vi "Initialize_Kate_Module.vi"(8 "Error In":errorcluster, 11 "UI Controls Refnum":T1) -> (0 "Error Out":errorcluster)   [LabVIEW 2012]
doc: "SciScan 1.2 160622"
uses:
  Custom Control and Typedefs/UI Controls Refnum.ctl
  Custom Control and Typedefs/ChannelSelector_for_PosSave.ctl
  Custom Controls/PositionSaveMod.ctl
  Custom Control and Typedefs/Overlay Control.ctl
  CommonResource VIs/UI Control and Indicator properties_Commands.ctl
  Image Validity FGV_Commands.ctl
  Custom Controls/MAIN Image panel tab Control type def.ctl
  Custom Controls/MAIN Image panel reso tab Control type def.ctl
  Chnl_2_tab_Commands.ctl
  GFG/GFG library.lvlib
panel:
  # "Red (Current Image)"
  # "Green (Saved Image)"
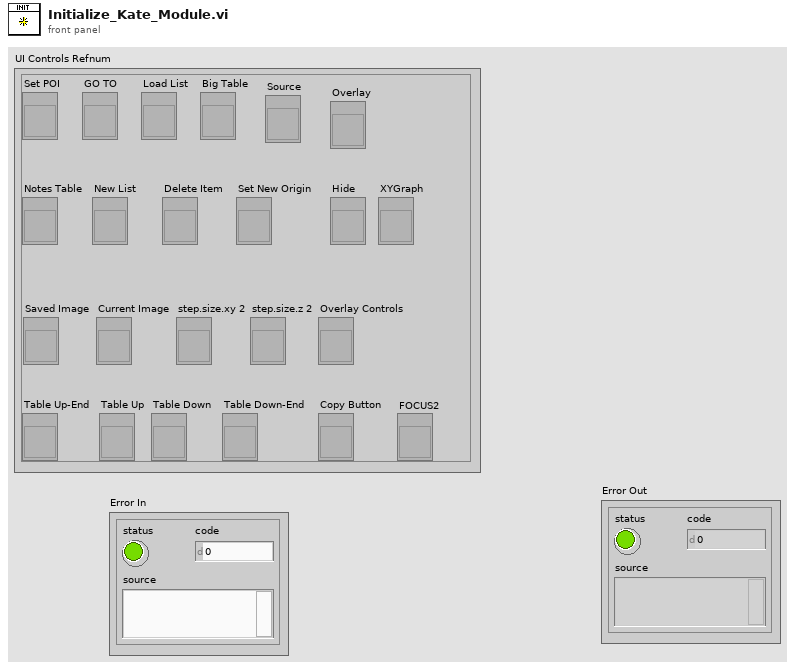
[diagram p1: front panel]
types:
  T1 = typedef "UI Controls Refnum.ctl" = cluster{"GO TO":refnum<vi>, "Load List":refnum<vi>, "Big Table":refnum<vi>, "Notes Table":refnum<vi>, "New List":refnum<vi>, "Delete Item":refnum<vi>, "Set New Origin":refnum<vi>, "Set POI":refnum<vi>, "Saved Image":refnum<vi>, "Current Image":refnum<vi>, "step.size.xy 2":refnum<vi>, "step.size.z 2":refnum<vi>, "Source":refnum<vi>, "Table Up-End":refnum<vi>, "Table Up":refnum<vi>, "Table Down":refnum<vi>, "Table Down-End":refnum<vi>, "Copy Button":refnum<vi>, "Hide":refnum<vi>, "Overlay Controls":refnum<vi>, "Overlay":refnum<vi>, "XYGraph":refnum<vi>, "FOCUS2":refnum<vi>}
  T2 = typedef "Image Validity FGV_Commands.ctl" = enum16{"Set validity status", "Get Validity status"}
  T3 = typedef "UI Control and Indicator properties_Commands.ctl" = enum16{"Enable", "Disable", "Disable and Grey", "Make Visible", "Make Invisible"}
  T4 = typedef "Chnl_2_tab_Commands.ctl" = enum16{"ChannelToTab", "TabToChannel"}
  T5 = typedef "MAIN Image panel reso tab Control type def.ctl" = enum32{"Channel 1", "Channel 2", "Channel 3", "Channel 4", "Channel 5", "all channels", "RGB overlay", "ROI", "arbitrary line scan"}
  T6 = typedef "MAIN Image panel tab Control type def.ctl" = enum32{"Channel 1", "Channel 2", "Channel 3", "Channel 4", "all channels", "RGB overlay", "ROI", "arbitrary line scan"}
  T7 = typedef "ChannelSelector_for_PosSave.ctl" = enum16{"Channel 1", "Channel 2", "Channel 3", "Channel 4"}
  T8 = cluster{"WaveformChartRef":refnum<vi>, "DigitalRef":refnum<vi>, "ArrayRef":refnum<vi>, "TabControlRef":refnum<vi>, "EnumRef":refnum<vi>, "RingRef":refnum<vi>, "BooleanRef":refnum<vi>, "KnobRef":refnum<vi>, "SlideRef":refnum<vi>, "PathRef":refnum<vi>, "StringRef":refnum<vi>, "ComboBox":refnum<vi>, "WaveformGraphRef":refnum<vi>}
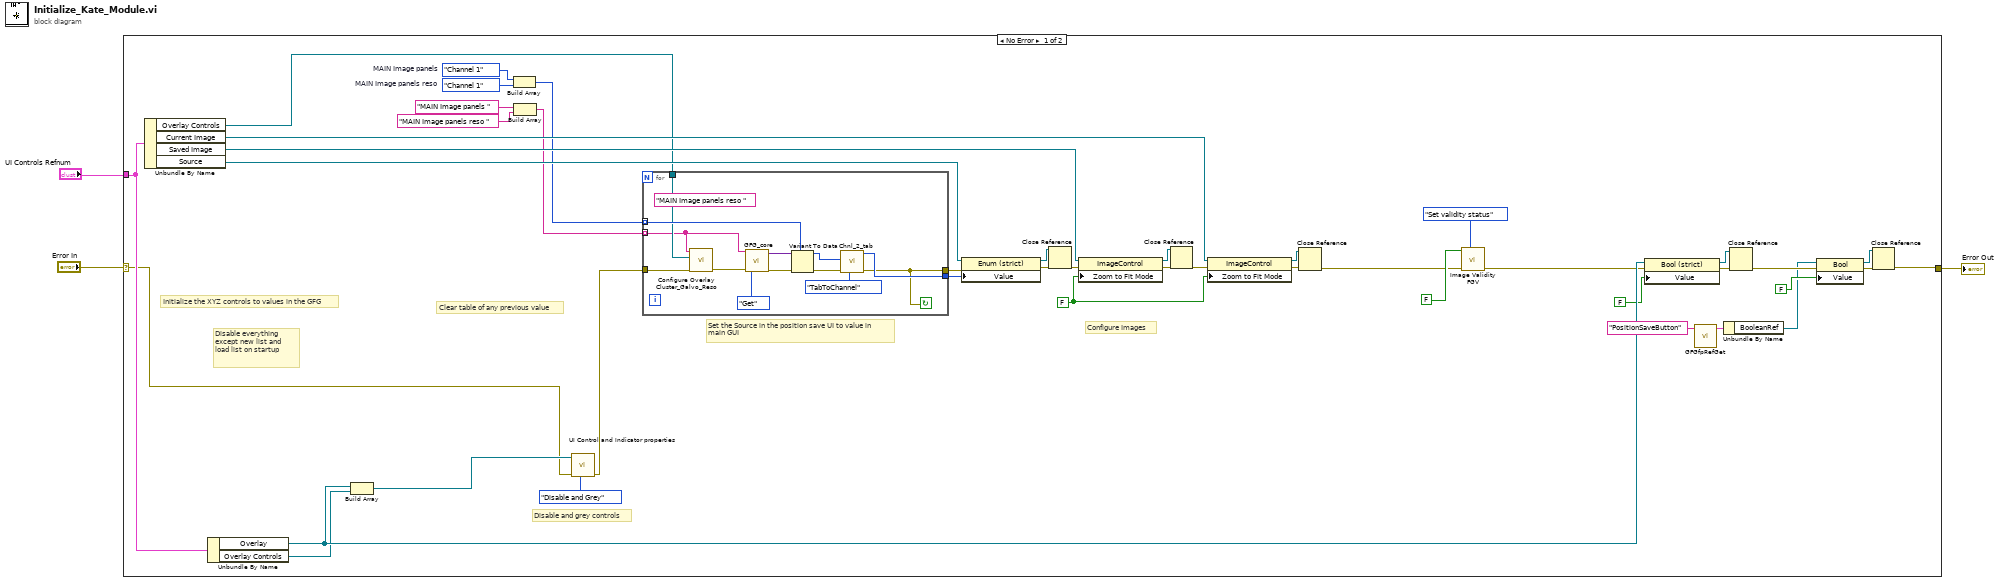
[diagram p0: block diagram]
diagram:
  n1 = case shown="No Error" "Error In" {
    selector: "Error In" -> [w7 w60]
    tunnel: "UI Controls Refnum" -> [w30 _]
    tunnel: [w9 w60] -> w1
    frame No Error {
      w18 = MAIN_Image_panel_reso_tab_Control_type_def."Channel 1"  # MAIN Image panels reso
      w19 = MAIN_Image_panel_tab_Control_type_def."Channel 1"  # MAIN Image panels
      w43 = FALSE ("Zoom to Fit Mode")
      # "Disable and grey controls"
      # "Clear table of any previous value"
      # "Disable everything except new list and load list on startup"
      # "Configure Images"
      # "Set the Source in the position save UI to value in \nmain GUI"
      # "Initialize the XYZ controls to values in the GFG"
      n2 = Unbundle By Name(w30) -> ("Overlay Controls"=w8:refnum<vi>, "Current Image"=w38:refnum<vi>, "Saved Image"=w39:refnum<vi>, "Source"=w44:refnum<vi>)
      n3 = Unbundle By Name(w30) -> ("Overlay"=w24:refnum<vi>, "Overlay Controls"=w20:refnum<vi>)
      n4 = Build Array(w24, w20) -> (w32:refnum<vi>[])
      n5 = Build Array(w19, w18) -> (w17:u32[])
      n6 = Build Array("MAIN Image panels " ("Variable Name in"), "MAIN Image panels reso " ("Variable Name in")) -> (w27:string[])
      n7 = call "UI Control and Indicator properties.vi"("Enable Command"=UI_Control_and_Indicator_properties_Commands."Disable and Grey", "Error In"=w7, "Control Refnums"=w32) -> ("Error Out"=w5:errorcluster)  [unwired: 8 in]
      n8 = for {
        tunnel: [w57] -> w46
        tunnel: [w51] -> w45
        tunnel: w5 -> [w50]
        tunnel: w27 -> [w47] mode=indexing
        tunnel: w17 -> [w52] mode=indexing
        tunnel: w8 -> [w48]
        stop <- w51 continue-if-true
        (unwired) "MAIN Image panels reso " ("Variable Name in")
        n9 = call "Configure Overlay Cluster_Galvo_Reso.vi"("Error In"=w50, "Overlay Control Reference"=w48, "Overlay Control Type"=w47) -> ("Error Out"=w49:errorcluster)  [unwired: 8 in]
        n10 = call "GFG_core.vi"("Variable Name in"=w47, "error in (no error)"=w49, "Action"=enum16{"Init", "Set", "Get"}."Get") -> ("Variant Out"=w59:variant, "error out"=w58:errorcluster)  [unwired: 10 in, 5 out]
        n11 = Variant To Data(error in=w58, type=w52, Variant=w59) -> (data=w53:u32, error out=w55:errorcluster)
        n12 = call "Chnl_2_tab.vi"("Command"=Chnl_2_tab_Commands."TabToChannel", "Error In"=w55, "Tab IN"=w53) -> ("Error Out"=w51:errorcluster, "Channel  OUT"=w57:T7)  [unwired: 6 in, 1 out]
      }
      n13 = property on="Property Node" class="Enum (strict)"(reference=w44, error in=w45, "Value"=w46) -> (reference out=w41:refnum<vi>, error out=w42:errorcluster)
      n14 = Close Reference(reference=w41, error in (no error)=w42) -> (error out=w40:errorcluster)
      n15 = property class="ImageControl"(reference=w39, error in=w40, "Zoom to Fit Mode"=w43) -> (reference out=w36:refnum<vi>, error out=w37:errorcluster)
      n16 = Close Reference(reference=w36, error in (no error)=w37) -> (error out=w33:errorcluster)
      n17 = property class="ImageControl"(reference=w38, error in=w33, "Zoom to Fit Mode"=w43) -> (reference out=w34:refnum<vi>, error out=w35:errorcluster)
      n18 = Close Reference(reference=w34, error in (no error)=w35) -> (error out=w6:errorcluster)
      n19 = call "Image Validity FGV.vi"("Image Validity FGV_Commands"=Image_Validity_FGV_Commands."Set validity status", "Error In"=w6, "Validity status IN"=FALSE) -> ("Error Out"=w4:errorcluster)  [unwired: 7 in, 1 out]
      n20 = property class="Bool (strict)"(reference=w24, error in=w4, "Value"=FALSE) -> (reference out=w21:refnum<vi>, error out=w23:errorcluster)
      n21 = call "GFGfpRefGet.vi"("Variable Name in"="PositionSaveButton") -> ("output cluster"=w15:T8)  [unwired: 9 in, 1 out]
      n22 = Unbundle By Name(w15) -> ("BooleanRef"=w12:refnum<vi>)
      n23 = Close Reference(reference=w21, error in (no error)=w23) -> (error out=w14:errorcluster)
      n24 = property class="Bool"(reference=w12, error in=w14, "Value"=FALSE) -> (reference out=w10:refnum<vi>, error out=w11:errorcluster)
      n25 = Close Reference(reference=w10, error in (no error)=w11) -> (error out=w9:errorcluster)
    }
    frame Error {
    }
  }
  "Error Out" <- w1
